vi "svfa_Three Finger Peak Search.vi"(2 "FFT Size":i32=512, 3 "window length":i32=512, 4 "window":T1(ring), 5 "three fingers":dbl[](array[numeric]) format="%.6e") -> (0 "freq":dbl format="%.6f", 1 "amplitude":dbl format="%.2f")   [LabVIEW 2017]
uses:
  <vilib>/addons/_NISVFA/_Spectrum Processing/subVIs/svfa_Rect Window Frequency Response.vi
  <vilib>/addons/_NISVFA/_Spectrum Processing/subVIs/svfa_Cosine Window Coefficients.vi
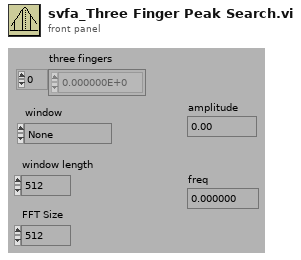
[diagram p1: front panel]
types:
  T1 = enum16{"None ", "Hanning", "Hamming", "Blackman-Harris", "Exact Blackman", "Blackman", "Flat Top", "4 Term B-Harris ", "7 Term B-Harris", "Low Sidelobe"}
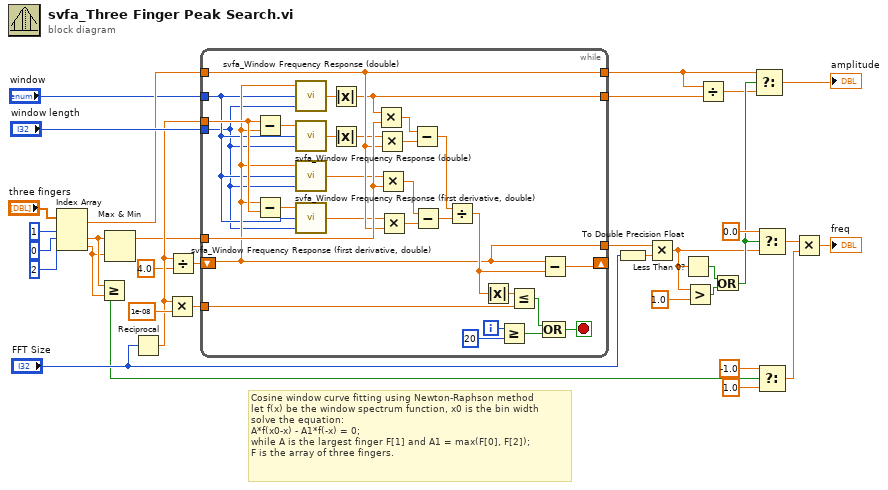
[diagram p0: block diagram]
diagram:
  # "Cosine window curve fitting using Newton-Raphson method\nlet f(x) be the window spectrum function, x0 is the bin width\nsolve the equation:\nA*f(x0-x) - A1*f(-x) = 0;\nwhile A is the largest finger F[1] and A1 = max(F[0], F[2]);\nF is the array of three fingers."
  n1 = Index Array(array="three fingers", index #1=1 ("Index"), index #2=0 ("Index"), index #3=2 ("Index")) -> (element #1=w24:dbl, element #2=w3:dbl, element #3=w1:dbl)
  n2 = Greater Or Equal?(x=w3, y=w1) -> (x >= y?=w5:bool)
  n3 = Max & Min(x=w3, y=w1) -> (max(x,y)=w7:dbl)  [unwired: 1 out]
  n4 = Reciprocal(x="FFT Size") -> (1/x=w28:dbl)
  n5 = Multiply(x=w28, y=1e-08) -> (x*y=w30:dbl)
  n6 = Divide(x=w28, y=4.0) -> (x/y=w29:dbl)
  n7 = while {
    tunnel: [w42] -> w10
    tunnel: [w45] -> w23
    tunnel: [w52] -> w14
    tunnel: w24 -> [w52]
    tunnel: w30 -> [w47]
    tunnel: w7 -> [w55]
    tunnel: w28 -> [w53]
    tunnel: "window length" -> [w39]
    tunnel: "window" -> [w40]
    shift-left: w29 -> [w42]
    shift-right: [w46] -> _
    i -> [w63]
    stop <- w49 stop-if-true
    n8 = Subtract(x=w53, y=w42) -> (x-y=w43:dbl)
    n9 = Subtract(x=w42, y=w53) -> (x-y=w41:dbl)
    n10 = call <vilib>:"svfa_Window Frequency Response (double).vi"("N (window length)"=w39, "window"=w40, "f(normalized)"=w42) -> ("H(f)"=w38:cdb)
    n11 = call <vilib>:"svfa_Window Frequency Response (double).vi"("N (window length)"=w39, "window"=w40, "f(normalized)"=w43) -> ("H(f)"=w37:cdb)
    n12 = call <vilib>:"svfa_Window Frequency Response (first derivative, double).vi"("N (window length)"=w39, "window"=w40, "f(normalized)"=w42) -> ("H'(f)"=w36:dbl)
    n13 = call <vilib>:"svfa_Window Frequency Response (first derivative, double).vi"("N (window length)"=w39, "window"=w40, "f(normalized)"=w41) -> ("H'(f)"=w35:dbl)
    n14 = Absolute Value(x=w38) -> (abs(x)=w45:dbl)
    n15 = Absolute Value(x=w37) -> (abs(x)=w44:dbl)
    n16 = Multiply(x=w45, y=w55) -> (x*y=w61:dbl)
    n17 = Multiply(x=w44, y=w52) -> (x*y=w60:dbl)
    n18 = Multiply(x=w36, y=w55) -> (x*y=w59:dbl)
    n19 = Multiply(x=w35, y=w52) -> (x*y=w58:dbl)
    n20 = Subtract(x=w61, y=w60) -> (x-y=w51:dbl)
    n21 = Subtract(x=w59, y=w58) -> (x-y=w57:dbl)
    n22 = Divide(x=w51, y=w57) -> (x/y=w54:dbl)
    n23 = Absolute Value(x=w54) -> (abs(x)=w56:dbl)
    n24 = Greater Or Equal?(x=w63, y=20) -> (x >= y?=w50:bool)
    n25 = Less Or Equal?(x=w56, y=w47) -> (x <= y?=w48:bool)
    n26 = Subtract(x=w42, y=w54) -> (x-y=w46:dbl)
    n27 = Compound Arithmetic op=OR(w48, w50) -> (w49:bool)
  }
  n28 = To Double Precision Float(number="FFT Size") -> (double precision float=w9:dbl)
  n29 = Multiply(x=w10, y=w9) -> (x*y=w11:dbl)
  n30 = Less Than 0?(x=w11) -> (x < 0?=w21:bool)
  n31 = Greater?(x=w11, y=1.0) -> (0:w20:bool)
  n32 = Divide(x=w14, y=w23) -> (x/y=w15:dbl)
  n33 = Or(x=w21, y=w20) -> (x .or. y?=w16:bool)
  n34 = Select(t=w14, s=w16, f=w15) -> (s? t:f=→"amplitude":dbl)
  n35 = Select(t=0.0, s=w16, f=w11) -> (s? t:f=w18:dbl)
  n36 = Select(t=-1.0, s=w5, f=1.0) -> (s? t:f=w12:dbl)
  n37 = Multiply(x=w18, y=w12) -> (x*y=→"freq":dbl)
